vi "ConvertHexStringToAsciiStr.vi"(11 "hex string":string) -> (3 "ascii string":string)   [LabVIEW 2018, in "Library-DataConvert.lvlib"]
uses:
  Library-DataConvert.lvlib
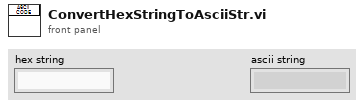
[diagram p1: front panel]
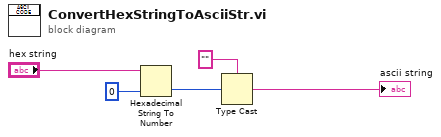
[diagram p0: block diagram]
diagram:
  n1 = Hexadecimal String To Number(string="hex string", default (0uL)=u8 0) -> (number=w5:u8)  [unwired: 1 in, 1 out]
  n2 = Type Cast(type="", x=w5) -> (*(type *) &x=→"ascii string":string)
